vi "Autonomous Independent.vi"   [LabVIEW 2013]
doc: "This VI is called when autonomous begins, and will automatically be terminated when autonomous ends. You can carry out timed or sensor driven robot movement independently without needing to return to the caller."
uses:
  Autonomous States.ctl
  <vilib>/Rock Robotics/WPI/Solenoid/WPI_SolenoidValue.ctl
  Robot Global Data.vi
  <vilib>/Rock Robotics/WPI/RobotDrive/WPI_RobotDriveGetSetRefNum.vi
  <vilib>/Rock Robotics/WPI/Solenoid/WPI_SolenoidSetEnum.vi
  <vilib>/Rock Robotics/WPI/RobotDrive/WPI_RobotDriveArcadeDrive_Standard(NoSaturation).vi
  <vilib>/addons/control/pid/pid.llb/PID (DBL).vi
  <vilib>/Rock Robotics/WPI/Joystick/WPI_JoystickGetSetRefNum.vi
  <vilib>/addons/control/pid/NI_PID_pid.lvlib
panel:
  # "Be sure to right-click and choose Data Operations>>Make Current Value default if you want to save the array values with the VI"
types:
  T1 = typedef "Autonomous States.ctl" = enum16{"init", "arms down", "drive", "wait", "shoot", "stop"}
  T2 = typedef "WPI_JoystickDevRef.ctl" = cluster{"Device":T3}
  T3 = typedef "WPI_JoystickDeviceEnum.ctl" = enum16{"USB 1", "USB 2", "USB 3", "USB 4", "Kinect 1", "Kinect 2"}
  T4 = cluster{"axis 1 (x)":dbl, "axis 2 (y)":dbl, "axis 3 (throttle)":dbl, "axis 4":dbl, "axis 5":dbl, "axis 6":dbl}
  T5 = typedef "WPI_GyroDevRef.ctl" = cluster{"DevStatus":errorcluster, "Analog Module":T6, "Analog Channel":T7, "Offset":dbl, "Gain (VoltsPerDegree/Second)":dbl}
  T6 = typedef "FPGA_TypedefAnalogModule.ctl" = enum16{"Analog Module 1", "Analog Module 2"}
  T7 = typedef "FPGA_AIChannel.ctl" = enum8{"AI 1", "AI 2", "AI 3", "AI 4", "AI 5", "AI 6", "AI 7", "AI 8", "Invalid"}
  T8 = typedef "WPI_EncoderDevRef.ctl" = cluster{"DevStatus":errorcluster, "EncoderIndex":T9, "CounterIndex":T10, "DistancePerCount":dbl, "Decoding Type":T11}
  T9 = typedef "FPGA_EncoderIdx.ctl" = enum8{"Enc 0", "Enc 1", "Enc 2", "Enc 3", "Invalid"}
  T10 = typedef "FPGA_CounterCtrSystemIndex.ctl" = enum8{"Ctr 0", "Ctr 1", "Ctr 2", "Ctr 3", "Ctr 4", "Ctr 5", "Ctr 6", "Ctr 7", "Invalid"}
  T11 = typedef "WPI_EncoderType.ctl" = enum16{"1x", "2x", "4x"}
  T12 = typedef "WPI_SolenoidDevRef.ctl" = cluster{"DevStatus":errorcluster, "Solenoid Module":T13, "Forward Solenoid Channel":T14, "Reverse Solenoid Channel":T14}
  T13 = typedef "FPGA_TypedefSolenoidModule.ctl" = enum16{"Solenoid Module 1", "Solenoid Module 2"}
  T14 = typedef "WPI_SolenoidChannel.ctl" = enum8{"Solenoid 1", "Solenoid 2", "Solenoid 3", "Solenoid 4", "Solenoid 5", "Solenoid 6", "Solenoid 7", "Solenoid 8", "Invalid"}
  T15 = typedef "WPI_RobotDriveDevRef.ctl" = cluster{"DevStatus":errorcluster, "Motors[]":T16[], "Square Inputs":bool, "Max Output":dbl, "Isochronous":bool}
  T16 = typedef "WPI_MotorControlDeviceRef.ctl" = cluster{"DeviceStatus":errorcluster, "Type":enum16{"PWM", "CAN"}, "PWM":cluster{"Digital Module":T17, "PWM Channel":T18, "DeadBand":T19}, "CAN":cluster{"Device Number":u8, "Control Mode":T20, "Semaphore":T21, "Max Vout":dbl}, "Invert":bool, "TransformRef":T22, "InvTransformRef":T22}
  T17 = typedef "FPGA_TypedefDigitalModule.ctl" = enum16{"Digital Module 1", "Digital Module 2"}
  T18 = typedef "FPGA_DIOPWMChannel.ctl" = enum8{"PWM 1", "PWM 2", "PWM 3", "PWM 4", "PWM 5", "PWM 6", "PWM 7", "PWM 8", "PWM 9", "PWM 10", "Invalid"}
  T19 = typedef "WPI_PWMDeadband.ctl" = cluster{"Name":string, "maxPositivePwm":i32, "minPositivePwm":i32, "centerPwm":i32, "maxNegativePwm":i32, "minNegativePwm":i32, "angularRange":u16}
  T20 = typedef "WPI_CANJaguar_ControlMode.ctl" = enum8{"Percent VBus", "Current", "Speed", "Position", "Voltage"}
  T21 = typedef "Semaphore RefNum" = refnum<k1>
  T22 = typedef "WPI_PWMTransform_ConPane.ctl" = refnum<vi>
  T23 = typedef "WPI_SolenoidValue.ctl" = enum16{"Off", "On", "Forward", "Reverse"}
  T24 = cluster{"proportional gain (Kc)":dbl, "integral time (Ti, min)":dbl, "derivative time (Td, min)":dbl}
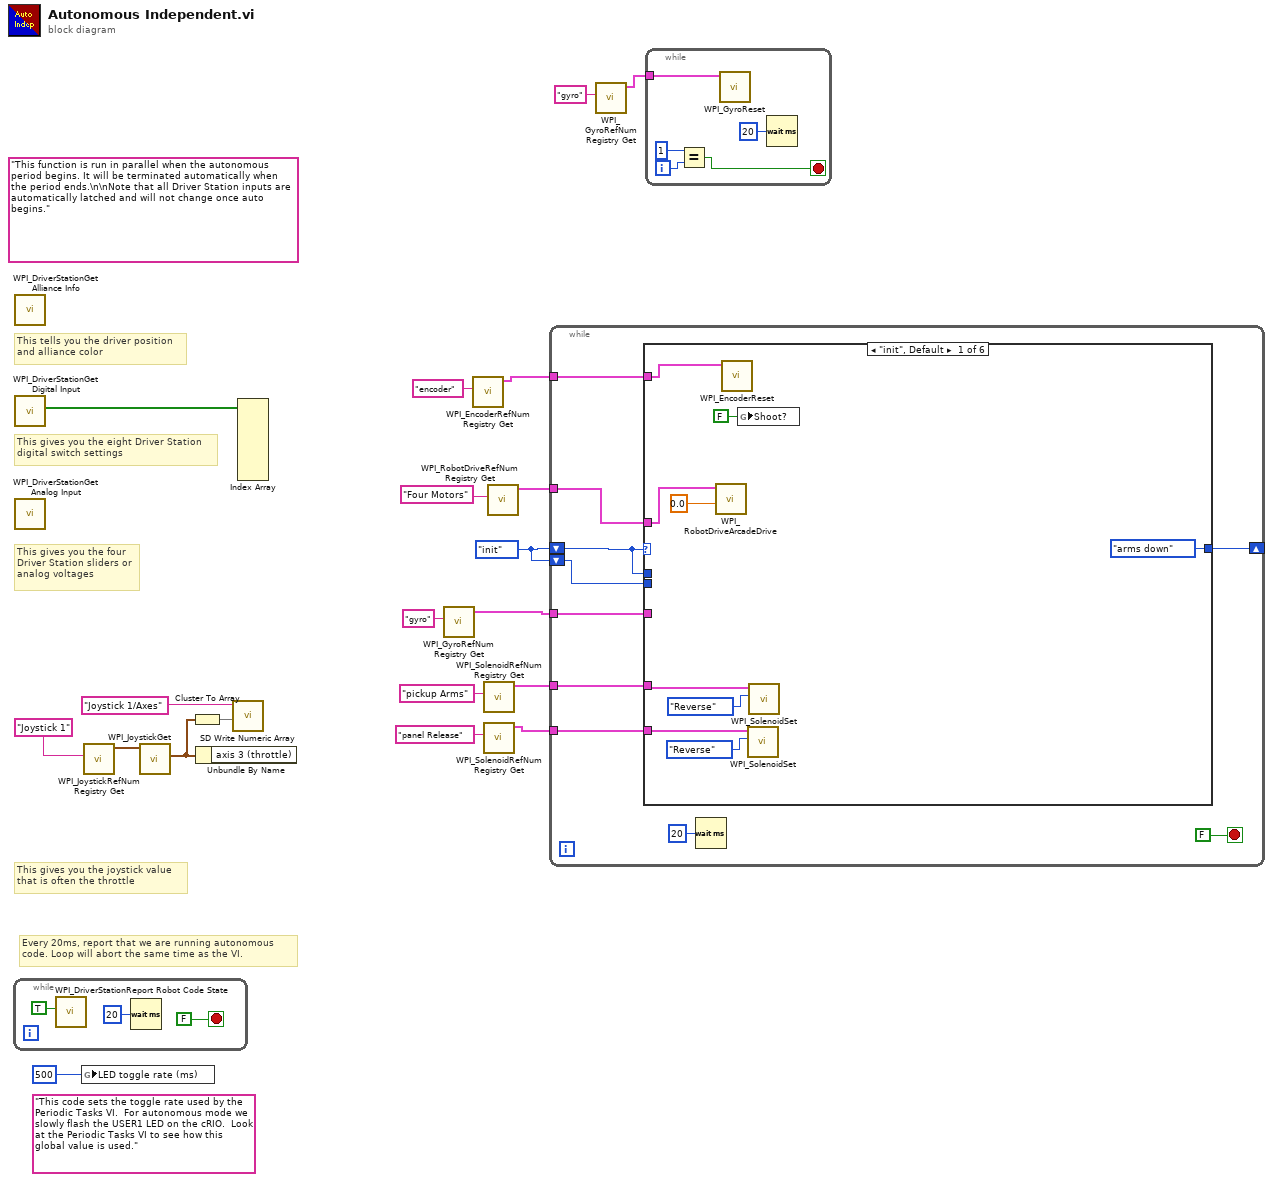
[diagram p0: block diagram]
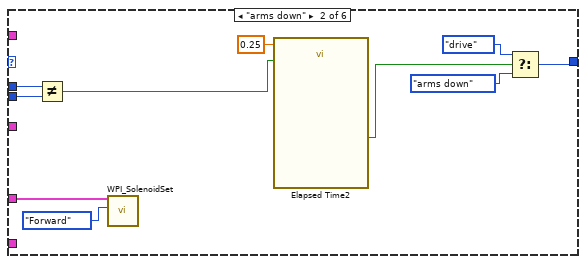
[diagram p2: hidden frame]
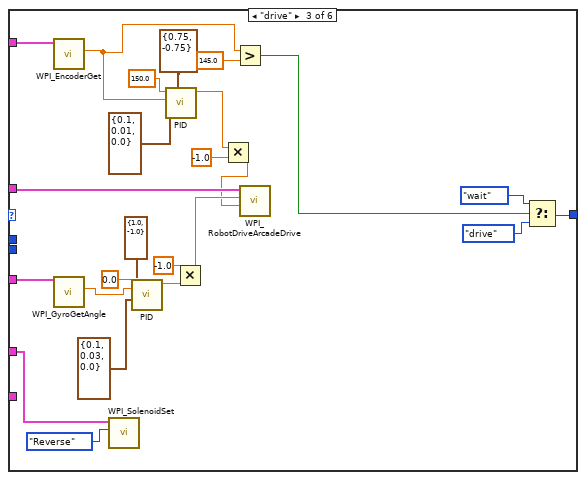
[diagram p3: hidden frame]
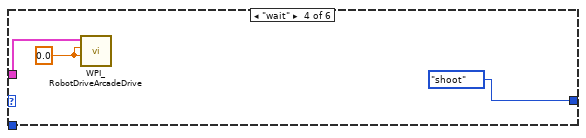
[diagram p4: hidden frame]
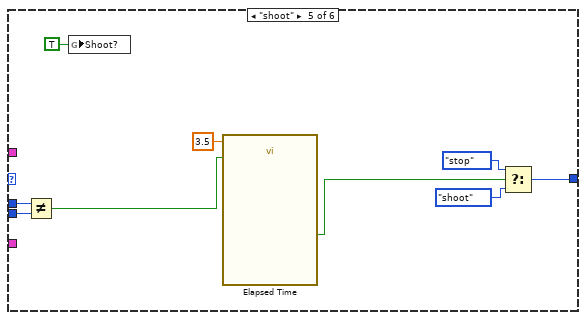
[diagram p5: hidden frame]
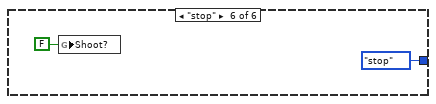
[diagram p6: hidden frame]
diagram:
  w7 = Autonomous_States."init"
  (unwired) "This code sets the toggle rate used by the Periodic Tasks VI.  For autonomous mode we slowly flash the USER1 LED on the cRIO.  Look at the Periodic Tasks VI to see how this global value is used."
  (unwired) "This function is run in parallel when the autonomous period begins. It will be terminated automatically when the period ends.\n\nNote that all Driver Station inputs are automatically latched and will not change once auto begins."
  # "Every 20ms, report that we are running autonomous\ncode. Loop will abort the same time as the VI."
  # "This gives you the joystick value\nthat is often the throttle"
  # "This tells you the driver position\nand alliance color"
  # "This gives you the eight Driver Station\ndigital switch settings"
  # "This gives you the four\nDriver Station sliders or\nanalog voltages"
  n1 = while {
    stop <- FALSE stop-if-true
    n2 = call <vilib>:"WPI_DriverStationReport Robot Code State.vi"("Autonomous"=TRUE) -> ()  [unwired: 10 in, 1 out]
    n3 = Wait (ms)(milliseconds to wait=u32 20) -> ()  [unwired: 1 out]
  }
  n4 = call <vilib>:"WPI_DriverStationGet Alliance Info.vi"() -> ()  [unwired: 12 out]
  n5 = call <vilib>:"WPI_DriverStationGet Digital Input.vi"() -> ("Driver Station Digital Input (1-8)"=w20:bool[])  [unwired: 11 out]
  n6 = call <vilib>:"WPI_DriverStationGet Analog Input.vi"() -> ()  [unwired: 12 out]
  n7 = global write "Robot Global Data.vi" "LED toggle rate (ms)"(u32 500 ("LED ms toggle rate")) -> ()
  n8 = call <vilib>:"WPI_JoystickRefNum Registry Get.vi"("refnum name"="Joystick 1") -> ("JoystickDevRef"=w18:T2)  [unwired: 1 in, 9 out]
  n9 = call <vilib>:"WPI_JoystickGet.vi"("JoystickDevRef"=w18) -> ("Axes"=w15:T4)  [unwired: 1 in, 5 out]
  n10 = Cluster To Array(cluster=w15) -> (array=w16:dbl[])
  n11 = Unbundle By Name(w15) -> ()  [unwired: 1 out]
  n12 = call <vilib>:"SD Write Numeric Array.vi"("Numeric Array"=w16, "Name"="Joystick 1/Axes") -> ()  [unwired: 8 in, 2 out]
  n13 = Index Array(array=w20) -> ()  [unwired: 8 in, 8 out]
  n14 = call <vilib>:"WPI_GyroRefNum Registry Get.vi"("refnum name"="gyro") -> ("GyroDevRef"=w10:T5)  [unwired: 9 in, 1 out]
  n15 = call <vilib>:"WPI_EncoderRefNum Registry Get.vi"("refnum name"="encoder") -> ("EncoderDevRef"=w5:T8)  [unwired: 9 in, 1 out]
  n16 = call <vilib>:"WPI_SolenoidRefNum Registry Get.vi"("refnum name"="pickup Arms") -> ("SolenoidDevRef"=w3:T12)  [unwired: 9 in, 1 out]
  n17 = call <vilib>:"WPI_SolenoidRefNum Registry Get.vi"("refnum name"="panel Release") -> ("SolenoidDevRef"=w1:T12)  [unwired: 9 in, 1 out]
  n18 = call <vilib>:"WPI_RobotDriveRefNum Registry Get.vi"("refnum name"="Four Motors") -> ("RobotDriveDevRef"=w12:T15)  [unwired: 9 in, 1 out]
  n19 = while {
    shift-right: [w32] -> _
    shift-left: w7 -> [w28]
    tunnel: w12 -> [w33]
    tunnel: w10 -> [w29]
    shift-left: w7 -> [w26]
    tunnel: w5 -> [w27]
    tunnel: w3 -> [w25]
    tunnel: w1 -> [w24]
    stop <- FALSE stop-if-true
    n20 = case shown="\"init\", Default" w28 {
      tunnel: w33 -> [w42 _ w76 w79 _ _]
      tunnel: [Autonomous_States."arms down" w47 w73 Autonomous_States."shoot" w83 Autonomous_States."stop"] -> w32
      tunnel: w29 -> [_ _ w72 _ _ _]
      tunnel: w28 -> [_ w45 _ _ w82 _]
      tunnel: w27 -> [w34 _ w64 _ _ _]
      tunnel: w26 -> [_ w44 _ _ w81 _]
      tunnel: w25 -> [w38 w52 w54 _ _ _]
      tunnel: w24 -> [w35 _ _ _ _ _]
      frame "init", Default {
        n21 = call-poly <vilib>:"WPI_RobotDriveArcadeDrive.vi"("Y axis value"=0.0, "RobotDriveDevRef"=w42) -> ()  [unwired: 7 in, 3 out]
        n22 = call <vilib>:"WPI_EncoderReset.vi"("EncoderDevRef"=w34) -> ()  [unwired: 9 in, 2 out]
        n23 = global write "Robot Global Data.vi" "Shoot?"(FALSE ("Shoot?")) -> ()
        n24 = call-poly <vilib>:"WPI_SolenoidSet.vi"("Value"=WPI_SolenoidValue."Reverse", "SolenoidDevRef"=w35) -> ()  [unwired: 8 in, 2 out]
        n25 = call-poly <vilib>:"WPI_SolenoidSet.vi"("Value"=WPI_SolenoidValue."Reverse", "SolenoidDevRef"=w38) -> ()  [unwired: 8 in, 2 out]
      }
      frame "arms down" {
        n26 = Not Equal?(x=w45, y=w44) -> (x != y?=w43:bool)
        n27 = call-poly <vilib>:"WPI_SolenoidSet.vi"("Value"=WPI_SolenoidValue."Forward", "SolenoidDevRef"=w52) -> ()  [unwired: 8 in, 2 out]
        n28 = call "Elapsed Time2"("Time Target (s)"=0.25, "Reset"=w43) -> ("Time has Elapsed"=w50:bool)  [unwired: 10 in, 7 out]
        n29 = Select(t=Autonomous_States."drive", s=w50, f=Autonomous_States."arms down") -> (s? t:f=w47:T1)
      }
      frame "drive" {
        n30 = call <vilib>:"WPI_EncoderGet.vi"("EncoderDevRef"=w64) -> ("Distance"=w59:dbl)  [unwired: 5 in, 5 out]
        n31 = call <vilib>:"WPI_GyroGetAngle.vi"("GyroDevRef"=w72) -> ("Angle"=w70:dbl)  [unwired: 7 in, 3 out]
        n32 = call-poly <vilib>:"WPI_SolenoidSet.vi"("Value"=WPI_SolenoidValue."Reverse", "SolenoidDevRef"=w54) -> ()  [unwired: 8 in, 2 out]
        n33 = call-poly <vilib>:"PID.vi"("output range"=cluster{"output high":dbl, "output low":dbl} {"output high"=1.0, "output low"=-1.0}, "PID gains"=T24 {"proportional gain (Kc)"=0.1, "integral time (Ti, min)"=0.03, "derivative time (Td, min)"=0.0}, "process variable"=w70, "setpoint"=0.0) -> ("output"=w67:dbl)  [unwired: 6 in, 1 out]
        n34 = call-poly <vilib>:"PID.vi"("output range"=cluster{"output high":dbl, "output low":dbl} {"output high"=0.75, "output low"=-0.75}, "PID gains"=T24 {"proportional gain (Kc)"=0.1, "integral time (Ti, min)"=0.01, "derivative time (Td, min)"=0.0}, "process variable"=w59, "setpoint"=150.0) -> ("output"=w57:dbl)  [unwired: 6 in, 1 out]
        n35 = Multiply(x=-1.0, y=w67) -> (x*y=w71:dbl)
        n36 = Multiply(x=w57, y=-1.0) -> (x*y=w62:dbl)
        n37 = Greater?(x=w59, y=145.0) -> (0:w63:bool)
        n38 = call-poly <vilib>:"WPI_RobotDriveArcadeDrive.vi"("Y axis value"=w62, "X axis value"=w71, "RobotDriveDevRef"=w76) -> ()  [unwired: 6 in, 3 out]
        n39 = Select(t=Autonomous_States."wait", s=w63, f=Autonomous_States."drive") -> (s? t:f=w73:T1)
      }
      frame "wait" {
        w78 = 0.0 ("Y axis value")
        n40 = call-poly <vilib>:"WPI_RobotDriveArcadeDrive.vi"("Y axis value"=w78, "X axis value"=w78, "RobotDriveDevRef"=w79) -> ()  [unwired: 6 in, 3 out]
      }
      frame "shoot" {
        n41 = Not Equal?(x=w82, y=w81) -> (x != y?=w80:bool)
        n42 = global write "Robot Global Data.vi" "Shoot?"(TRUE ("Shoot?")) -> ()
        n43 = call "Elapsed Time"("Time Target (s)"=3.5, "Reset"=w80) -> ("Time has Elapsed"=w86:bool)  [unwired: 10 in, 7 out]
        n44 = Select(t=Autonomous_States."stop", s=w86, f=Autonomous_States."shoot") -> (s? t:f=w83:T1)
      }
      frame "stop" {
        n45 = global write "Robot Global Data.vi" "Shoot?"(FALSE ("Shoot?")) -> ()
      }
    }
    n46 = Wait (ms)(milliseconds to wait=u32 20) -> ()  [unwired: 1 out]
  }
  n47 = call <vilib>:"WPI_GyroRefNum Registry Get.vi"("refnum name"="gyro") -> ("GyroDevRef"=w8:T5)  [unwired: 9 in, 1 out]
  n48 = while {
    tunnel: w8 -> [w92]
    i -> [w95]
    stop <- w93 stop-if-true
    n49 = Equal?(x=1, y=w95) -> (x = y?=w93:bool)
    n50 = call <vilib>:"WPI_GyroReset.vi"("GyroDevRef"=w92) -> ()  [unwired: 9 in, 2 out]
    n51 = Wait (ms)(milliseconds to wait=u32 20) -> ()  [unwired: 1 out]
  }
